vi "TPG261_Info.vi"(8 "error in (no error)":errorcluster caption="Fehler (Eingang, kein Fehler)", 11 "input refnum":refnum<visa-resource-name> caption="ComPort") -> (0 "error out":errorcluster, 3 "ComPort out":refnum<visa-resource-name>, 4 "SP1-Params":string, 5 "gaugeStatus":string, 7 "gaugeID":string)   [LabVIEW 2012]
doc: "This VI is an example of how to use the PV ActiveLine subVIs programmatically. This VI first initializes the instrument, takes measurements, then closes the instrument."
uses:
  <instrlib>/PV ActiveLine/PV ActiveLine.lvlib
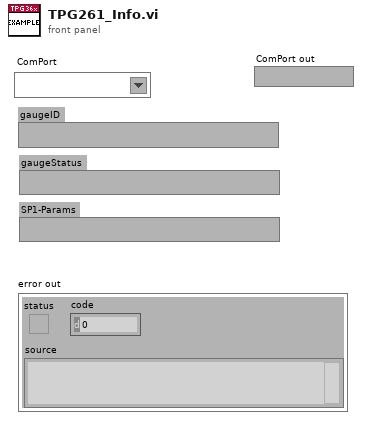
[diagram p1: front panel]
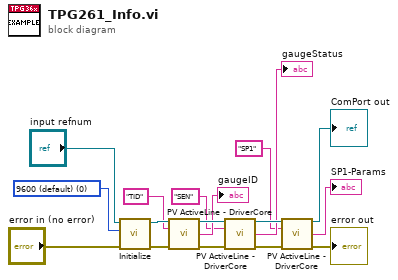
[diagram p0: block diagram]
diagram:
  w15 = u32 0 items=["9600 (default)", "19200", "38400", "57600", "115200"] ("Baud Rate")
  n1 = call <instrlib>:"Initialize.vi"("error in (no error)"="error in (no error)", "Baud Rate"=w15, "input refnum"="input refnum") -> ("Cluster (Ausgang)"=w14:errorcluster, "Referenz out"=w13:refnum<visa-resource-name>)  [unwired: 7 in]
  n2 = call <instrlib>:"PV ActiveLine - DriverCore.vi"("Referenz in"=w13, "Command"="TID", "Fehler (Eingang)"=w14) -> ("Referenz out"=w12:refnum<visa-resource-name>, "String Out"=→"gaugeID":string, "Cluster (Ausgang)"=w11:errorcluster)  [unwired: 10 in]
  n3 = call <instrlib>:"PV ActiveLine - DriverCore.vi"("Referenz in"=w12, "Command"="SEN", "Fehler (Eingang)"=w11) -> ("Referenz out"=w10:refnum<visa-resource-name>, "String Out"=→"gaugeStatus":string, "Cluster (Ausgang)"=w9:errorcluster)  [unwired: 10 in]
  n4 = call <instrlib>:"PV ActiveLine - DriverCore.vi"("Referenz in"=w10, "Command"="SP1", "Fehler (Eingang)"=w9) -> ("Referenz out"=→"ComPort out":refnum<visa-resource-name>, "String Out"=→"SP1-Params":string, "Cluster (Ausgang)"=→"error out":errorcluster)  [unwired: 10 in]
